vi "AlliGator Use Phasor Graph Selected Phasor Plots Principal Axis - UC Intersections as References.vi"(7 "Selected Plot List":string, 8 "error in (no error)":errorcluster, 9 "Major Axis?":bool, 10 "Selected Plot Indices":i32[](array[numeric]), 11 "Phasor Graph refnum":refnum<vi>) -> (0 "error out":errorcluster, 1 "Message":string, 2 "Intersection 1":cluster{"x":dbl, "y":dbl}, 3 "Intersection 2":cluster{"x":dbl, "y":dbl})   [LabVIEW 2021, in "AlliGator Phasor Graph.lvlib"]
doc: "Defines references as the intersection of the major or minor axis of inertia of the phasor plot with the UC."
uses:
  AlliGator Phasor Graph.lvlib
  576fdb66-777c-4f0c-9114-c95863eebee2.vi
  Utilities/Logical Processors Used.vi
  Phasor/Phasor.lvlib
  Math/Math.lvlib
panel:
  # "see the AlliGator License on the block diagram (Ctrl+E or Window:Show Block Diagram)"
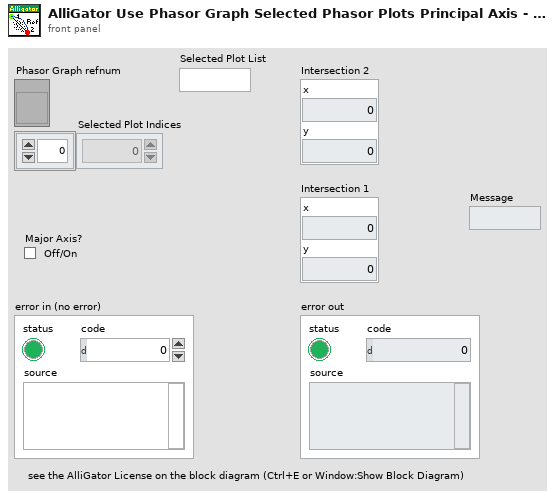
[diagram p1: front panel]
types:
  T1 = typedef "Phasor.lvlib/Phasor (g, s).ctl" = cluster{"g":dbl, "s":dbl}
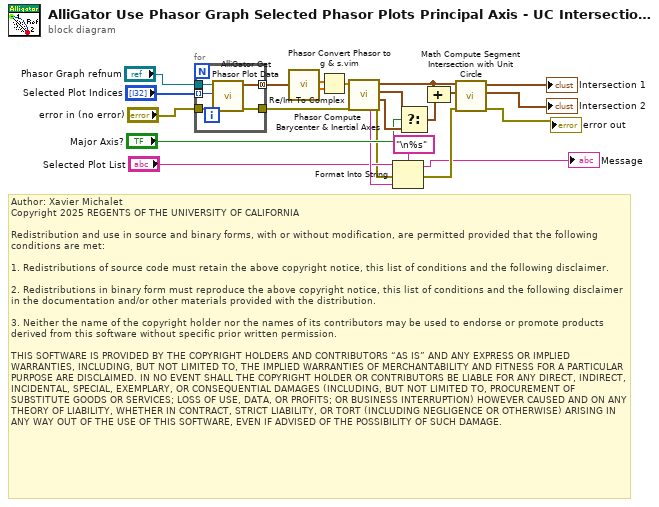
[diagram p0: block diagram]
diagram:
  # "Author: Xavier Michalet\nCopyright 2025 REGENTS OF THE UNIVERSITY OF CALIFORNIA\n\nRedistribution and use in source and binary forms, with or without modification, are permitted provided that the following conditions are met:\n\n1. Redistributions of source code must retain the above copyright notice, this list of conditions and the following disclaimer.\n\n2. Redistributions in binary form must reproduce the above copyright notice, this list of conditions and the following disclaimer in the documentation and/or other materials provided with the distribution.\n\n3. Neither the name of the copyright holder nor the names of its contributors may be used to endorse or promote products derived from this software without specific prior written permission.\n\nTHIS SOFTWARE IS PROVIDED BY THE COPYRIGHT HOLDERS AND CONTRIBUTORS “AS IS” AND ANY EXPRESS OR IMPLIED WARRANTIES, INCLUDING, BUT NOT LIMITED TO, THE IMPLIED WARRANTIES OF MERCHANTABILITY AND FITNESS FOR A PARTICULAR PURPOSE ARE DISCLAIMED. IN NO EVENT SHALL THE COPYRIGHT HOLDER OR CONTRIBUTORS BE LIABLE FOR ANY DIRECT, INDIRECT, INCIDENTAL, SPECIAL, EXEMPLARY, OR CONSEQUENTIAL DAMAGES (INCLUDING, BUT NOT LIMITED TO, PROCUREMENT OF SUBSTITUTE GOODS OR SERVICES; LOSS OF USE, DATA, OR PROFITS; OR BUSINESS INTERRUPTION) HOWEVER CAUSED AND ON ANY THEORY OF LIABILITY, WHETHER IN CONTRACT, STRICT LIABILITY, OR TORT (INCLUDING NEGLIGENCE OR OTHERWISE) ARISING IN ANY WAY OUT OF THE USE OF THIS SOFTWARE, EVEN IF ADVISED OF THE POSSIBILITY OF SUCH DAMAGE."
  n1 = for {
    tunnel: [w28] -> w1 mode=concatenating
    tunnel: "Phasor Graph refnum" -> [w26]
    tunnel: "error in (no error)" -> [w25]
    tunnel: [w27] -> w12
    tunnel: "Selected Plot Indices" -> [w24] mode=indexing
    n2 = call "AlliGator Get Phasor Plot Data.vi"("error in (no error)"=w25, "Plot Idx (-1: last)"=w24, "Phasor Graph Refnum"=w26) -> ("error out"=w27:errorcluster, "Phasor Array"=w28:T1[])  [unwired: 5 in, 2 out]
  }
  n3 = call "Phasor Convert Phasor to g & s.vim"("Phasor Array"=w1) -> ("g"=w15:dbl[], "s"=w14:dbl[])  [unwired: 8 in]
  n4 = Re/Im To Complex(1:w14, 2:w15) -> (0:w13:cdb[])
  n5 = call "Phasor Compute Barycenter & Inertial Axes.vi"("Error In"=w12, "Phasors"=w13) -> ("Error Out"=w5:errorcluster, "Minor Axis"=w17:cluster{"x":dbl, "y":dbl}, "Major Axis"=w18:cluster{"x":dbl, "y":dbl}, "Barycenter"=w20:cluster{"x":sgl, "y":sgl}, "Message"=w8:string)  [unwired: 5 in]
  n6 = Format Into String(format string="\n%s", initial string="Selected Plot List", error in=w5, w8) -> (resulting string=→"Message":string, error out=w4:errorcluster)
  n7 = Select(t=w18, s="Major Axis?", f=w17) -> (s? t:f=w16:cluster{"x":dbl, "y":dbl})
  n8 = Compound Arithmetic op=ADD(w20, w16) -> (w19:cluster{"x":dbl, "y":dbl})
  n9 = call "Math Compute Segment Intersection with Unit Circle.vi"("Error In"=w4, "Point 2"=w19, "Point 1"=w20) -> ("Error Out"=→"error out":errorcluster, "Intersection 2"=→"Intersection 2":cluster{"x1m":dbl, "y1m":dbl}, "Intersection 1"=→"Intersection 1":cluster{"x1p":dbl, "y1p":dbl})  [unwired: 6 in]
